vi "ModelConfigure.vi"(11 "Cluster in":refnum<vi>) -> (3 "Cluster out":refnum<vi>)   [LabVIEW 2013]
uses:
  <vilib>/Utility/error.llb/whitespace.ctl
  Control/Buffer.vi
  <vilib>/Utility/config.llb/Read Key (String).vi
  <vilib>/Utility/config.llb/NI_LVConfig.lvlib
panel:
  out "value":string
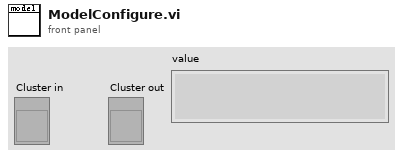
[diagram p1: front panel]
types:
  T1 = typedef "NI_LVConfig.lvlib/Config Data RefNum.ctl" = refnum<k1>
  T2 = typedef "whitespace.ctl" = u16
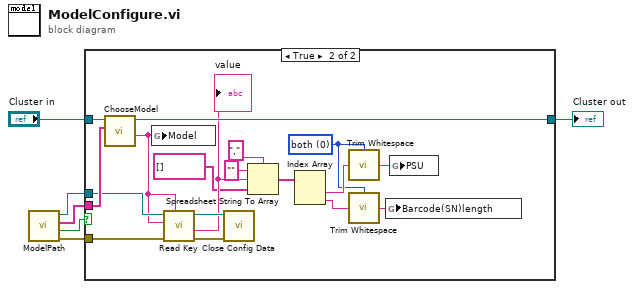
[diagram p0: block diagram]
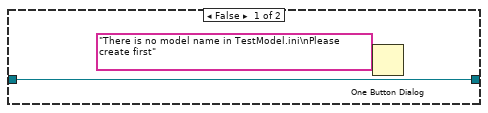
[diagram p2: hidden frame]
diagram:
  n1 = call "ModelPath.vi"() -> ("error out"=w2:errorcluster, "found?"=w4:bool, "Models"=w1:string[], "Refnum out"=w3:T1)  [unwired: 8 in]
  n2 = case shown="True" w4 {
    tunnel: "Cluster in" -> [w7 w25]
    tunnel: [w7 w24] -> w6
    tunnel: w1 -> [_ w26]
    tunnel: w3 -> [_ w23]
    tunnel: w2 -> [_ w22]
    frame False {
      n3 = One Button Dialog(message="There is no model name in TestModel.ini\nPlease create first") -> ()  [unwired: 1 in, 1 out]
    }
    frame True {
      w12 = T2 0 items=["both", "start of string", "end of string"] ("location (both)")
      n4 = call "ChooseModel.vi"("Array"=w26, "Information"=w25) -> ("Model"=w21:string, "Information"=w24:refnum<vi>)  [unwired: 8 in]
      n5 = global write "Buffer.vi" "Model"(w21) -> ()
      n6 = call-poly <vilib>:"Read Key.vi"("section"=w21, "error in (no error)"=w22, "key"=w21, "refnum"=w23) -> ("error out"=w19:errorcluster, "value"=w18:string, "refnum out"=w20:T1)  [unwired: 4 in, 1 out]
      "value" <- w18
      n7 = call <vilib>:"Close Config Data.vi"("error in (no error)"=w19, "refnum"=w20) -> ()  [unwired: 8 in, 2 out]
      n8 = Spreadsheet String To Array(delimiter (Tab)="," ("format string"), format string="", spreadsheet string=w18, array type (2D Dbl)=string[] []) -> (array=w17:string[])
      n9 = Index Array(array=w17) -> (element #1=w15:string, element #2=w9:string)  [unwired: 2 in]
      n10 = call <vilib>:"Trim Whitespace.vi"("string"=w15, "location (both)"=w12) -> ("trimmed string"=w14:string)
      n11 = call <vilib>:"Trim Whitespace.vi"("string"=w9, "location (both)"=w12) -> ("trimmed string"=w13:string)
      n12 = global write "Buffer.vi" "Barcode(SN)length"(w13) -> ()
      n13 = global write "Buffer.vi" "PSU"(w14) -> ()
    }
  }
  "Cluster out" <- w6
